vi "RenameGroupChannelTDMS.vi"(8 "error in (no error)":errorcluster, 11 "file path":path) -> (0 "error out":errorcluster)   [LabVIEW 2016]
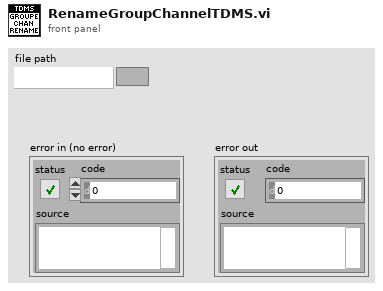
[diagram p1: front panel]
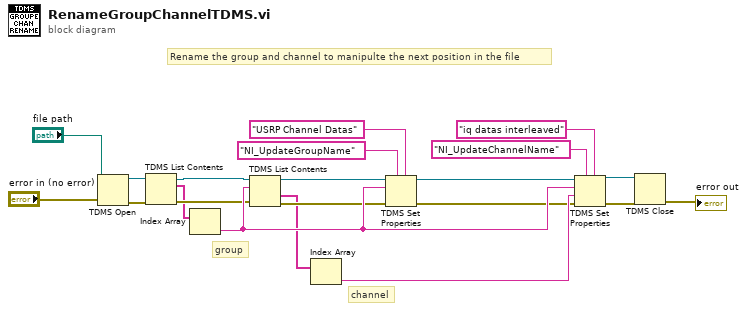
[diagram p0: block diagram]
diagram:
  # "Rename the group and channel to manipulte the next position in the file"
  # "channel"
  # "group"
  n1 = TDMS Open(8:"error in (no error)", 11:"file path") -> (0:w4:errorcluster, 3:w5:refnum<k34>)  [unwired: 5 in]
  n2 = TDMS List Contents(4:w4, 7:w5) -> (0:w11:errorcluster, 2:w8:string[], 3:w9:refnum<k34>)  [unwired: 1 in, 1 out]
  n3 = Index Array(array=w8) -> (element=w19:string)  [unwired: 1 in]
  n4 = TDMS List Contents(4:w11, 6:w19, 7:w9) -> (0:w15:errorcluster, 1:w10:string[], 3:w14:refnum<k34>)  [unwired: 1 out]
  n5 = Index Array(array=w10) -> (element=w20:string)  [unwired: 1 in]
  n6 = TDMS Set Properties(5:"USRP Channel Datas" ("element"), 7:"NI_UpdateGroupName" ("property names"), 8:w15, 10:w19, 11:w14) -> (0:w17:errorcluster, 3:w16:refnum<k34>)  [unwired: 1 in, 2 out]
  n7 = TDMS Set Properties(5:"iq datas interleaved" ("element"), 7:"NI_UpdateChannelName" ("property names"), 8:w17, 9:w20, 10:w19, 11:w16) -> (0:w3:errorcluster, 3:w1:refnum<k34>)  [unwired: 2 out]
  n8 = TDMS Close(8:w3, 11:w1) -> (0:→"error out":errorcluster)  [unwired: 1 out]
